vi "reciever_reading.vi"() -> ()   [LabVIEW 2021]
doc: "This template is for the Simple NI-USRP Streaming design, a design that shows the basics of streaming data to and from an NI USRP-294x/295x device. Refer to the block diagram for more information about how to use this template."
uses:
  Host/SubVIs/Start Trigger.ctl
  <vilib>/userDefined/Silver/nirio_resource_slv.ctl
  Host/SubVIs/Streaming Xvcr FPGA Ref.ctl
  Host/SubVIs/Initiate and Fetch (Multi).vi
  Host/SubVIs/Initiate and Fetch Time (Multi).vi
  Host/SubVIs/Initiate and Trigger.vi
  Host/SubVIs/Fetch Rx Data.vi
  Host/SubVIs/Fetch Rx Data (CDB WDT).vi
  Host/SubVIs/Check Aurora Link.vi
  Host/SubVIs/Check Stream Status.vi
  <vilib>/Utility/error.llb/Error Cluster From Error Code.vi
  <vilib>/rvi/errors/niLvFpgaAdjustHostInterfaceError.vi
  <vilib>/rvi/interface/nirviMethod/nirviMethod.xnode
  <vilib>/rvi/interface/nirviReadWriteControl/nirviReadWriteControl.xnode
  NiFpgaLv.dll
  <vilib>/rvi/interface/Simulation/niFpgaSimulationCallBeginRW.vi
  <vilib>/FPGAPlugInAG/Dynamic/niLvFpga_ReadFifo_Dynamic.vi
  <vilib>/rvi/errors/niLvFpgaMergeErrorWithErrorCode.vi
panel:
  out "IQ data overflow":u64
  in  "pre amp":dbl=15.0
  in  "Rx_detect_param":T1={"detection bar"=22.0, "max gap"=3, "max PW"=300, "min PW"=10} {"detection bar" format="%#_6p"}
  out "spots":i32
  in  "USRP RIO device":T2="RIO0" caption="USRP RIO Device"
  in  "start trigger":T3=enum."Immediate"
  out "acquiring":bool caption="Streaming"
  out "record time (ms)":u32
  out "write rate (SPS)":dbl format="%#_6p"
  out "write tdms loop time (ms)":u32
  in  "frequency":dbl=2000000000.0 format="%#_6p"
  in  "sample rate":dbl=10000000.0 format="%#_6p"
  out "get data loop time (ms)":u32 format="%.0p"
  out "error out":errorcluster
  in  "Stop":bool
  # "Overview: Demonstrates the use of the Advanced TDMS and simple streamer functions to write Rx data to a *.tdms file.\nInstructions:\nThis Vi must use Administrator privliges in order to write the data.\nthe USRP sohld be connected via MIXe to the computer (or other direct connection)\nset the params \nRun this VI.\ndue to the way the memory work after some time it can occer that the saveing rate will decrise."
  # "Rx Streaming"
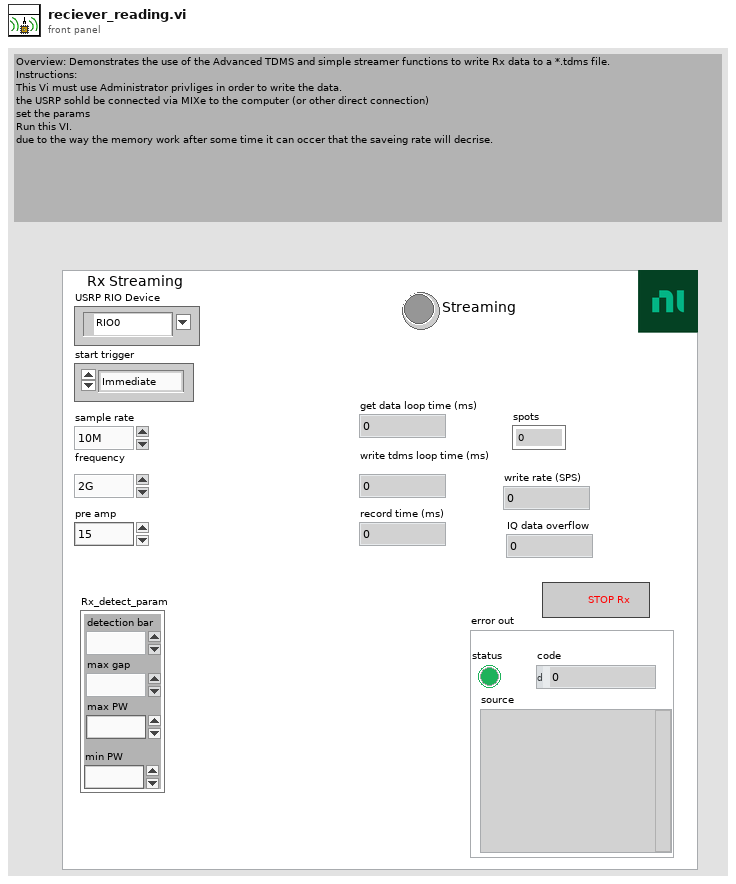
[diagram p1: front panel]
types:
  T1 = cluster{"detection bar":fxp<+,64,63>, "max gap":u8, "max PW":u16, "min PW":u16}
  T2 = typedef "nirio_resource_slv.ctl" = tag
  T3 = typedef "Start Trigger.ctl" = enum8{"Software", "Digital Edge", "Rx Start Trigger", "Tx Start Trigger", "Immediate", "Future Time Event"}
  T4 = cluster{"rf enable 0":bool, "rf config 0":cluster{"antenna":string, "frequency":dbl, "lo frequency":dbl, "level":dbl}, "rf enable 1":bool, "rf config 1":cluster{"antenna":string, "frequency":dbl, "lo frequency":dbl, "level":dbl}, "transfer mode":enum16{"Finite", "Continuous"}, "sample rate":dbl, "number of samples":u32, "start trigger":T3}
  T5 = enum16{"open", "open or create", "create or replace", "create", "open (read-only)"}
  T6 = typedef "Rx Channels.ctl" = cluster{"rx config":cluster{"channel configuration":cluster{"channel enable":bool, "channel configuration":cluster{"antenna":string, "frequency":dbl, "lo frequency":dbl, "level":dbl}}[], "transfer mode":enum16{"Finite", "Continuous"}, "sample rate":dbl, "number of samples":u32, "start trigger":T3}, "reference frequency source":string, "rx.data sink":enum16{"SFP Port 0", "SFP Port 1", "Host"}, "rx.enabled channels":string[], "vertical range":dbl[], "rx.coerced configurations":cluster{"coerced frequencies":dbl[], "coerced lo frequencies":dbl[], "coerced levels":dbl[], "coerced sample rates":dbl[]}}
  T7 = typedef "niUsrpRio Config v1 Host.lvlib/niUsrpRio Session.ctl" = cluster{"FPGA Interface":refnum<k20>, "RIO Interface Number":u32, "Data Clock Rate":u32, "FPGA Data Clock Rate":u32, "Global Settings Register Bus":T8, "Radio 0 Settings Register Bus":T8, "Radio 1 Settings Register Bus":T8, "Radio Settings Bus Semaphore":T9, "DB Queues":T10[], "Characterization Data Valid?":bool, "EEPROM Header":T11, "Device Data Header":T12, "EEPROM Characterization Header":T13, "Characterization Data":T14[], "FPGA Current Version":u32, "FPGA Oldest Compatible Version":u32, "Fixed Logic Current Version":u32, "Fixed Logic Oldest Compatible Version":u32, "FPGA Radio Settings Bus Current Version":u32, "FPGA Radio Settings Bus Oldest Compatible Version":u32, "FPGA Board Config Current Version":u32, "FPGA Board Config Oldest Compatible Version":u32, "Daughterboard Clock Rate":u32, "daughterboard configuration session handles":u64[]}
  T8 = typedef "niInstr Register Bus v0 Host.lvlib/Register Bus Session.ctl" = refnum<queue>
  T9 = typedef "Semaphore RefNum" = refnum<k1>
  T10 = typedef "niUsrpRio Config v1 Host.lvlib/DB Queue Reference.ctl" = refnum<queue>
  T11 = typedef "niUsrpRio Config v1 Host.lvlib/EEPROM Header.ctl" = cluster{"Checksum":u32, "Product Code":u16, "Hardware Current Version":u16, "Hardware Oldest Compatible Version":u16, "EEPROM Map Current Version":u16, "EEPROM Map Oldest Compatible Version":u16, "User Password":string, "Pointer to Factory Header":u32, "Pointer to User Header":u32, "Recommended Interval":u16, "Number of Reserved Bytes":i32, "Number of Daughterboards":u8, "Daughterboard IDs":u16[], "Daughterboard Serial Numbers":string[]}
  T12 = typedef "niUsrpRio Config v1 Host.lvlib/EEPROM Device Data Header.ctl" = cluster{"Checksum":u32, "Number of Channels":u8, "Number of Gain Settings":u16[], "Pointer to Characterization Data":u32[], "Number of Reserved Bytes":i32, "Number of Frequencies":u16[]}
  T13 = typedef "niUsrpRio Config v1 Host.lvlib/EEPROM Characterization Header.ctl" = cluster{"Checksum":u32, "Date":timestamp, "Temperature":sgl, "Misc. Info":string, "Pointer to Device Data Header":u32, "Number of Reserved Bytes":i32}
  T14 = typedef "niUsrpRio Config v1 Host.lvlib/Characterization Data.ctl" = cluster{"Gains[dB]":dbl[], "Frequencies [Hz]":dbl[], "IQ Imbalance Table":T15[], "Measured Gains[dB]":dbl[][]}
  T15 = typedef "niUsrpRio Config v1 Host.lvlib/IQ Imbalance.ctl" = cluster{"Gain Imbalance [linear]":dbl, "Phase Imbalance [radians]":dbl, "Offset":cdb}
  T16 = typedef "Streaming Xvcr FPGA Ref.ctl" = refnum<k20>
  T17 = cluster{"rx.state":enum16{"Idle", "Active"}, "rx.samples processed":u32, "rx.number of fifo overflows":u32, "rx.number of iq data overflows":u64[], "rx.dsp reset done":bool}
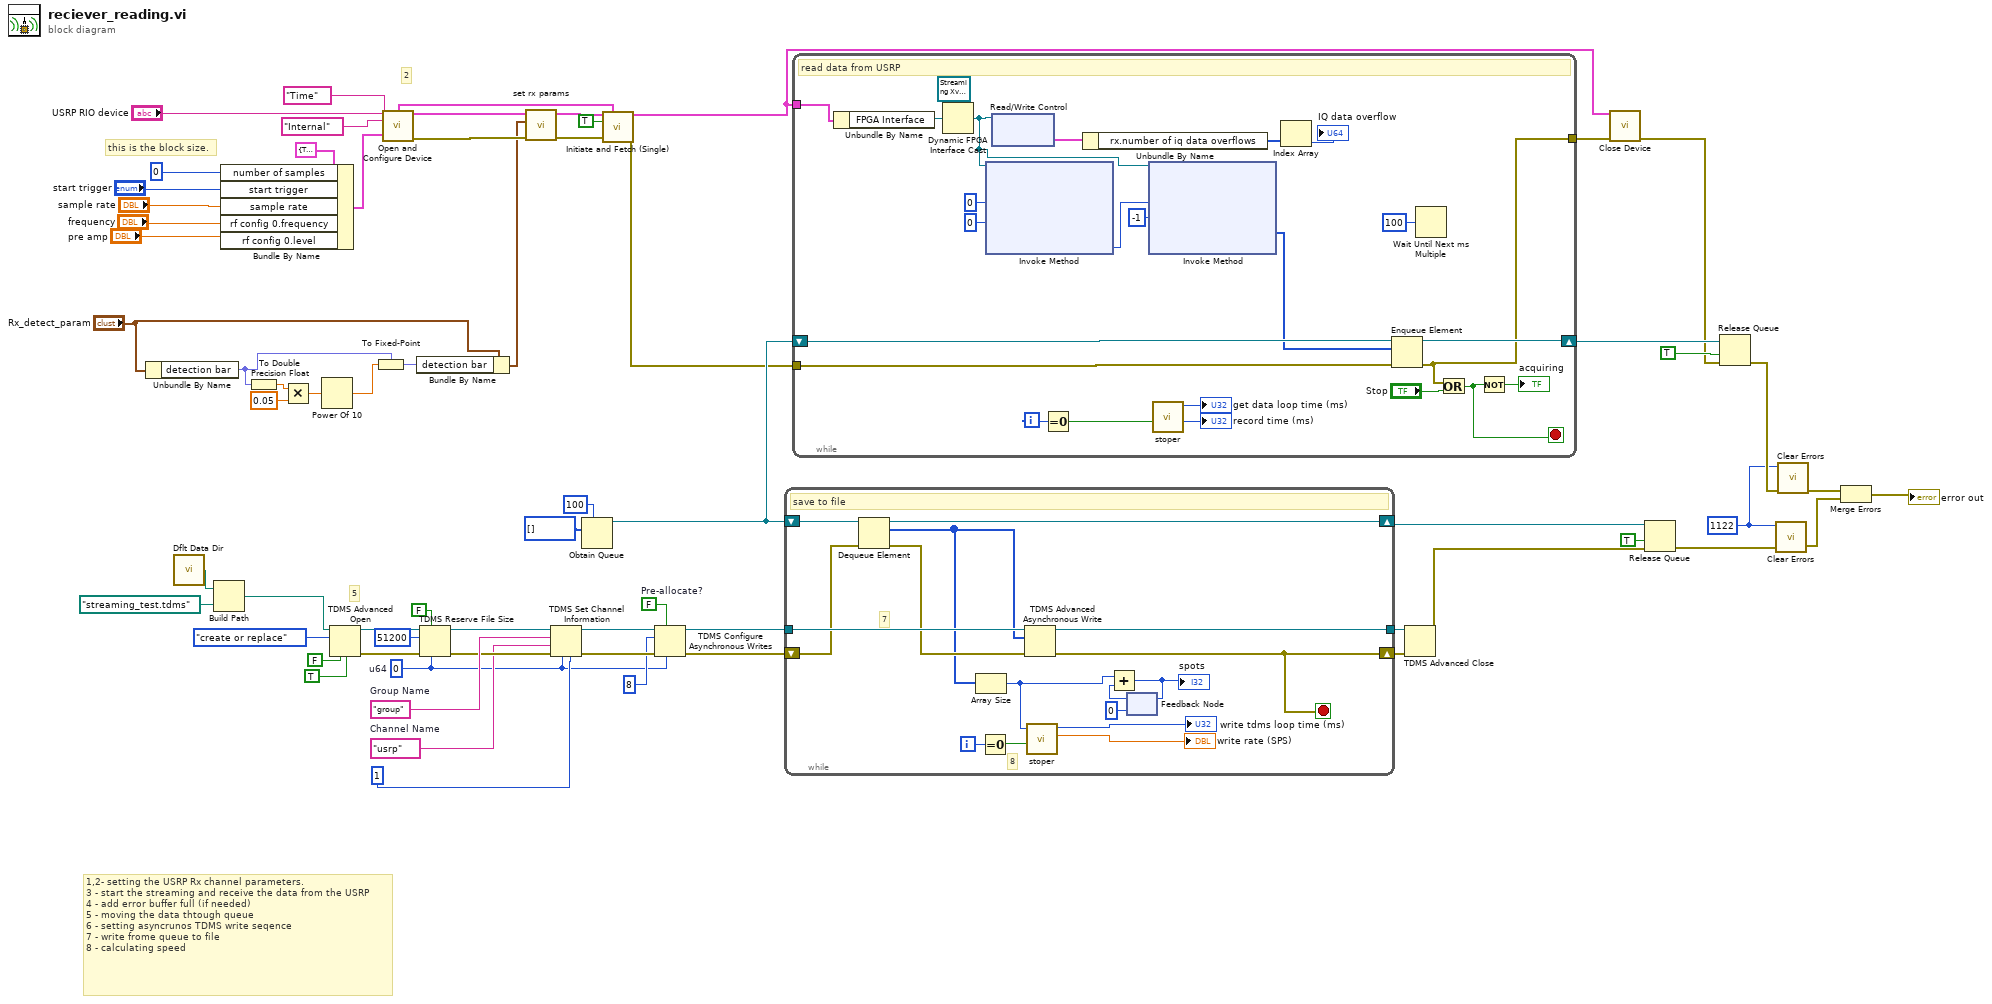
[diagram p0: block diagram]
diagram:
  w32 = 1122 ("specific error code to clear (0: all)")
  w57 = FALSE  # Pre-allocate?
  w48 = u64 0  # u64
  w66 = "group"  # Group Name
  w50 = "usrp"  # Channel Name
  # "2"
  # "this is the block size."
  # "1,2- setting the USRP Rx channel parameters.\n3 - start the streaming and receive the data from the USRP\n4 - add error buffer full (if needed)\n5 - moving the data thtough queue   \n6 - setting asyncrunos TDMS write seqence\n7 - write frome queue to file\n8 - calculating speed"
  # "5"
  n1 = Unbundle By Name("Rx_detect_param") -> ("detection bar"=w6:fxp<+,64,63>)
  n2 = call <vilib>:"Dflt Data Dir.vi"() -> ("App:Default Data Directory"=w43:path)
  n3 = Build Path(base path=w43, name or relative path=path "streaming_test.tdms") -> (appended path=w42:path)
  n4 = Bundle By Name(cluster=T4 {"rf enable 0"=TRUE, "rf config 0"={"antenna"="RX1", "frequency"=2000000000.0, "lo frequency"=-1.0, "level"=0.0}, "rf enable 1"=FALSE, "rf config 1"={"antenna"="RX2", "frequency"=2000000000.0, "lo frequency"=-1.0, "level"=0.0}, "transfer mode"=enum."Continuous", "sample rate"=10000000.0, "number of samples"=4194304, "start trigger"=enum."Immediate"} ("rx config"), "number of samples"=0, "start trigger"="start trigger", "sample rate"="sample rate", "rf config 0.frequency"="frequency", "rf config 0.level"="pre amp") -> (w24:T4)
  n5 = To Double Precision Float(number=w6) -> (double precision float=w5:dbl)
  n6 = Multiply(x=w5, y=0.05) -> (x*y=w3:dbl)
  n7 = Power Of 10(x=w3) -> (10^x=w2:dbl)
  n8 = TDMS Advanced Open(4:TRUE ("enable asynchronous? (T)"), 6:FALSE ("disable buffering? (T)"), 10:T5."create or replace" ("operation (0:open)"), 11:w42) -> (0:w62:errorcluster, 3:w63:refnum<k34>)  [unwired: 1 in, 1 out]
  n9 = To Fixed-Point(fixed-point type=w6, number=w2) -> (fixed-point=w1:fxp<+,64,63>)
  n10 = call "Open and Configure Device.vi"("USRP RIO Device"="USRP RIO device", "reference frequency source"="Internal", "which bitfile"="Time", "rx config"=w24) -> ("rx channels"=w13:T6, "niUsrpRio Session (out)"=w19:T7, "error out"=w18:errorcluster)  [unwired: 5 in, 4 out]
  n11 = Bundle By Name(cluster="Rx_detect_param", "detection bar"=w1) -> (w7:T1)
  n12 = TDMS Reserve File Size(6:w48, 7:FALSE ("append? (T)"), 8:w62, 10:u64 51200 ("reserve size"), 11:w63) -> (0:w60:errorcluster, 3:w61:refnum<k34>)
  n13 = call "set rx params.vi"("error in"=w18, "Rx_detect_param"=w7, "niUsrpRio Session (out)"=w19) -> ("error out"=w12:errorcluster, "niUsrpRio Session (out) 2"=w14:T7)  [unwired: 7 in]
  n14 = TDMS Set Channel Information(4:u32 1 ("y"), 6:w48, 8:w60, 9:w50, 10:w66, 11:w61) -> (0:w59:errorcluster, 3:w58:refnum<k34>)  [unwired: 1 in]
  n15 = Obtain Queue(max queue size (-1, unlimited)=100, element data type=u64[] [] ("waveform data")) -> (queue out=w33:refnum<queue>)  [unwired: 3 in, 2 out]
  n16 = call "Initiate and Fetch (Single).vi"("niUsrpRio Session"=w14, "rx channels"=w13, "first iteration"=TRUE, "error in"=w12) -> ("niUsrpRio Session (out)"=w11:T7, "error out"=w10:errorcluster)  [unwired: 9 in, 1 out]
  n17 = TDMS Configure Asynchronous Writes(6:w48, 7:w57, 8:w59, 10:u32 8 ("max asynchronous writes (4)"), 11:w58) -> (0:w51:errorcluster, 3:w54:refnum<k34>)  [unwired: 2 in]
  n18 = while {
    tunnel: w54 -> [w81]
    shift-right: [w76] -> w52
    shift-left: w33 -> [w82]
    tunnel: [w79] -> w53
    shift-right: [w80] -> w46
    shift-left: w51 -> [w75]
    i -> [w78]
    stop <- w80 stop-if-true
    # "8"
    # "7"
    # "save to file"
    n19 = Dequeue Element(queue=w82, error in (no error)=w75) -> (queue out=w76:refnum<queue>, element=w71:u64[], error out=w74:errorcluster)  [unwired: 1 in, 1 out]
    n20 = Array Size(array=w71) -> (size(s)=w70:i32)
    n21 = Equal To 0?(x=w78) -> (x = 0?=w73:bool)
    n22 = TDMS Advanced Asynchronous Write(8:w74, 10:w71, 11:w81) -> (0:w80:errorcluster, 3:w79:refnum<k34>)
    n23 = call "stoper.vi"("start"=w73, "x mission"=w70) -> ("x rate"=→"write rate (SPS)":dbl, "loop"=→"write tdms loop time (ms)":u32)  [unwired: 7 in, 1 out]
    n24 = feedback #1(0) -> (w68:i32)
    n25 = Add(x=w70, y=w68) -> (x+y=w69:i32)
    "spots" <- w69
    n26 = feedback-in #1(w69) -> ()
  }
  n27 = while {
    shift-right: [w106] -> w40
    shift-left: w33 -> [w105]
    tunnel: [w98] -> w22
    tunnel: w11 -> [w91]
    tunnel: w10 -> [w90]
    i -> [w99]
    stop <- w100 stop-if-true
    # "read data from USRP"
    n28 = Unbundle By Name(w91) -> ("FPGA Interface"=w96:refnum<k20>)
    n29 = Dynamic FPGA Interface Cast(Session In=T16 refnum ("Type"), Type=w96) -> (Session Out=w89:T16)
    n30 = xnode "Invoke Method"("FPGA VI Reference In"=w89, "Number of Elements"=u32 0, "Timeout (ms)"=0) -> ("Elements Remaining"=w88:u32)  [unwired: 1 in, 3 out]
    n31 = xnode "Read/Write Control"("FPGA VI Reference In"=w89) -> ("rx.status"=w94:T17)  [unwired: 1 in, 2 out]
    n32 = Equal To 0?(x=w99) -> (x = 0?=w97:bool)
    n33 = Unbundle By Name(w94) -> ("rx.number of iq data overflows"=w93:u64[])
    n34 = xnode "Invoke Method"("FPGA VI Reference In"=w89, "Number of Elements"=w88, "Timeout (ms)"=-1) -> ("Data"=w87:u64[])  [unwired: 1 in, 3 out]
    n35 = call "stoper.vi"("start"=w97) -> ("frome start"=→"record time (ms)":u32, "loop"=→"get data loop time (ms)":u32)  [unwired: 8 in, 1 out]
    n36 = Index Array(array=w93) -> (element=→"IQ data overflow":u64)  [unwired: 1 in]
    n37 = Enqueue Element(queue=w105, element=w87, error in (no error)=w90) -> (queue out=w106:refnum<queue>, error out=w98:errorcluster)  [unwired: 1 in, 1 out]
    n38 = Wait Until Next ms Multiple(millisecond multiple=u32 100) -> ()  [unwired: 1 out]
    n39 = Or(x=w98, y="Stop") -> (x .or. y?=w100:bool)
    n40 = Not(x=w100) -> (.not. x?=→"acquiring":bool)
  }
  n41 = TDMS Advanced Close(8:w46, 11:w53) -> (0:w41:errorcluster)  [unwired: 2 in, 1 out]
  n42 = call "Close Device.vi"("niUsrpRio Session"=w11, "error in"=w22) -> ("error out"=w23:errorcluster)  [unwired: 13 in]
  n43 = Release Queue(queue=w52, force destroy? (F)=TRUE, error in (no error)=w41) -> (error out=w34:errorcluster)  [unwired: 2 out]
  n44 = Release Queue(queue=w40, force destroy? (F)=TRUE, error in (no error)=w23) -> (error out=w35:errorcluster)  [unwired: 2 out]
  n45 = call <vilib>:"Clear Errors.vi"("error in (no error)"=w34, "specific error code to clear (0: all)"=w32) -> ("error out"=w31:errorcluster)  [unwired: 4 in, 1 out]
  n46 = call <vilib>:"Clear Errors.vi"("error in (no error)"=w35, "specific error code to clear (0: all)"=w32) -> ("error out"=w36:errorcluster)  [unwired: 4 in, 1 out]
  n47 = Merge Errors(w36, w31) -> (→"error out":errorcluster)
